vi "I2C Write.vi"(8 "error in (no error)":errorcluster, 9 "I2C Address (0x70)":i32=112 format="%x", 10 "Data":u8[](array[numeric])=[0] format="%x", 11 "I2C Task In":T1) -> (0 "error out":errorcluster, 3 "I2C Task Out":T1)   [LabVIEW 2017, in "I2C.lvlib"]
doc: "Writes the specified number of bytes from <b>Data</b> to the specified address. The I2C address is actually a 7-bit I2C address with an expansion of one 0 at the highest bit."
uses:
  <vilib>/robotics/Protocols/I2C/DAQmx/I2C.lvlib
  <vilib>/robotics/Protocols/I2C/DAQmx/Private/I2C Tasks.ctl
panel:
  # "The I2C address is actually a 7-bit I2C address with an expansion of one 0 at the highest bit."
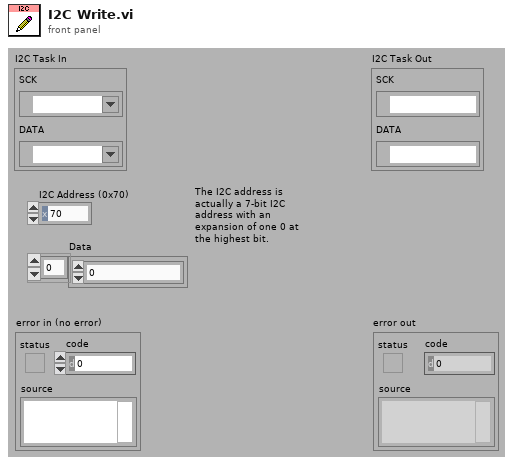
[diagram p1: front panel]
types:
  T1 = typedef "I2C.lvlib/I2C Tasks.ctl" = cluster{"SCK":refnum<k21>, "DATA":refnum<k21>}
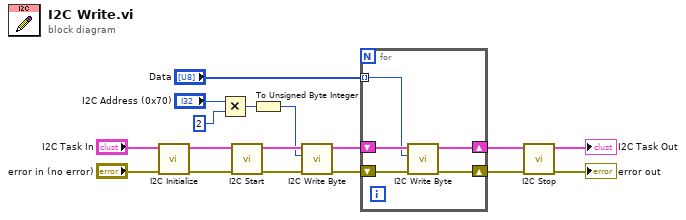
[diagram p0: block diagram]
diagram:
  n1 = call <vilib>:"I2C Initialize.vi"("error in (no error)"="error in (no error)", "I2C Task In"="I2C Task In") -> ("error out"=w14:errorcluster, "I2C Task Out"=w15:T1)  [unwired: 8 in]
  n2 = Multiply(x="I2C Address (0x70)", y=2) -> (x*y=w9:i32)
  n3 = call <vilib>:"I2C Start.vi"("error in (no error)"=w14, "I2C Task In"=w15) -> ("error out"=w12:errorcluster, "I2C Task Out"=w13:T1)  [unwired: 8 in]
  n4 = To Unsigned Byte Integer(number=w9) -> (unsigned 8bit integer=w8:u8)
  n5 = call <vilib>:"I2C Write Byte.vi"("error in (no error)"=w12, "Data Byte (0x0)"=w8, "I2C Task In"=w13) -> ("error out"=w5:errorcluster, "I2C Task Out"=w6:T1)  [unwired: 6 in, 1 out]
  n6 = for {
    tunnel: "Data" -> [w20] mode=indexing
    shift-right: [w19] -> w4
    shift-left: w6 -> [w22]
    shift-right: [w18] -> w3
    shift-left: w5 -> [w21]
    n7 = call <vilib>:"I2C Write Byte.vi"("error in (no error)"=w21, "Data Byte (0x0)"=w20, "I2C Task In"=w22) -> ("error out"=w18:errorcluster, "I2C Task Out"=w19:T1)  [unwired: 6 in, 1 out]
  }
  n8 = call <vilib>:"I2C Stop.vi"("error in (no error)"=w3, "I2C Task In"=w4) -> ("error out"=→"error out":errorcluster, "I2C Task Out"=→"I2C Task Out":T1)  [unwired: 8 in]
